vi "界面3子面板切换.vi"() -> ()   [LabVIEW 2013]
panel:
  in  "界面3子面板切换":i32
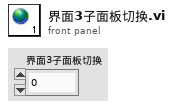
[diagram p1: front panel]
diagram:
